vi "Report Convert Date.vi"(11 "Date":string) -> (3 "result string":string)   [LabVIEW 2020, in "Report.lvlib"]
uses:
  Report.lvlib
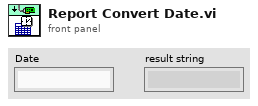
[diagram p1: front panel]
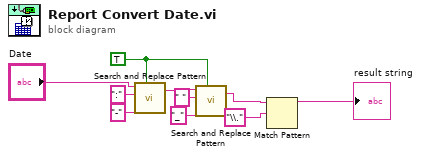
[diagram p0: block diagram]
diagram:
  w4 = TRUE ("replace all? (F)")
  n1 = call <vilib>:"Search and Replace Pattern.vi"("string"="Date", "regular expression (\"\")"=":" ("regular expression (\"\")"), "replace string (\"\")"="-" ("replace string (\"\")"), "replace all? (F)"=w4) -> ("result string"=w5:string)  [unwired: 1 in, 1 out]
  n2 = call <vilib>:"Search and Replace Pattern.vi"("string"=w5, "regular expression (\"\")"=" " ("regular expression (\"\")"), "replace string (\"\")"="_" ("replace string (\"\")"), "replace all? (F)"=w4) -> ("result string"=w3:string)  [unwired: 1 in, 1 out]
  n3 = Match Pattern(string=w3, regular expression="\\." ("replace string (\"\")")) -> (before substring=→"result string":string)  [unwired: 1 in, 3 out]
